vi "setup excel worksheet.vi"(0 "Current Sample Sheet":string="Sample 1", 1 "milliseconds to wait":u32=100, 3 "template file path":path=path "C:/Cascade/templates/Groundwater Profiling Log_empty_labview_template.xlsx", 4 "Excel report file path":path=path "C:/Cascade/Data/Excel Reports/Groundwater Profiling Log_ara1.xlsx", 5 "error in (no error)":errorcluster, 6 "Header path":path=path "C:/Cascade/templates/Fields for Excel sheets.xlsx", 7 "Open Excel Files":bool) -> (8 "subarray":string[][](array[string]), 10 "column max value":i32, 11 "row max value":i32, 12 "Column of Volume":i32, 13 "Worksheet Names":string[](array[string]), 14 "NI_report out":refnum<class "NI_report.lvclass">, 15 "Columns":i32[](array[numeric]), 16 "start of last occupied row":string, 17 "Number of Sample Sheets":i32, 18 "Select Worksheet Index":i32, 19 "error out":errorcluster)   [LabVIEW 2016]
uses:
  <vilib>/Utility/NIReport.llb/NI_report.lvclass
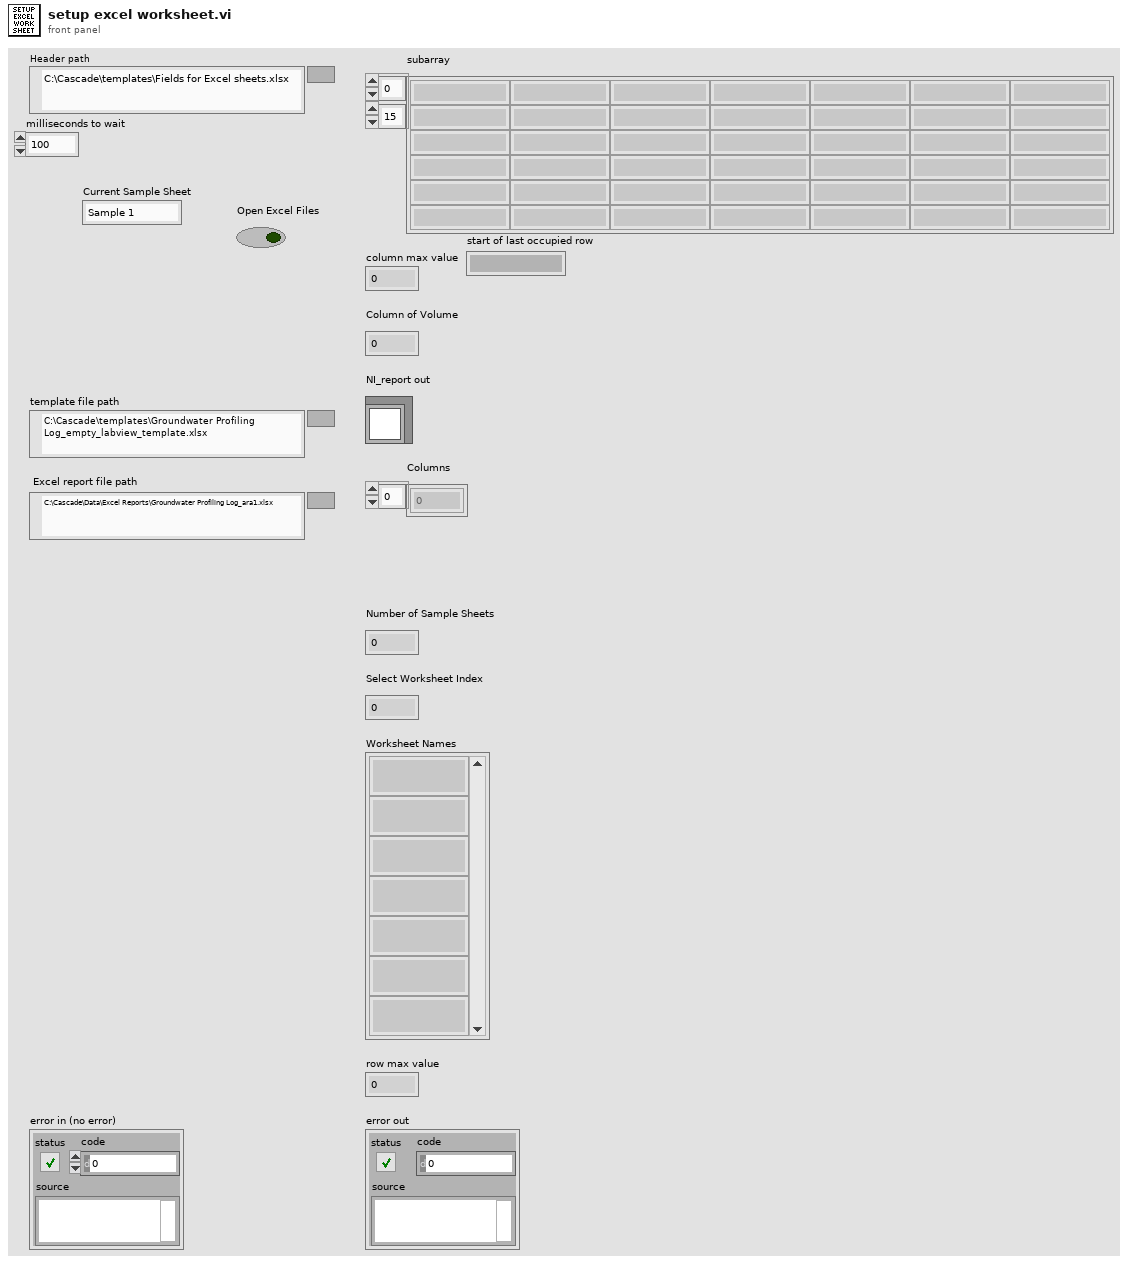
[diagram p1: front panel]
types:
  T1 = enum16{"maximized", "minimized", "normal", "no change"}
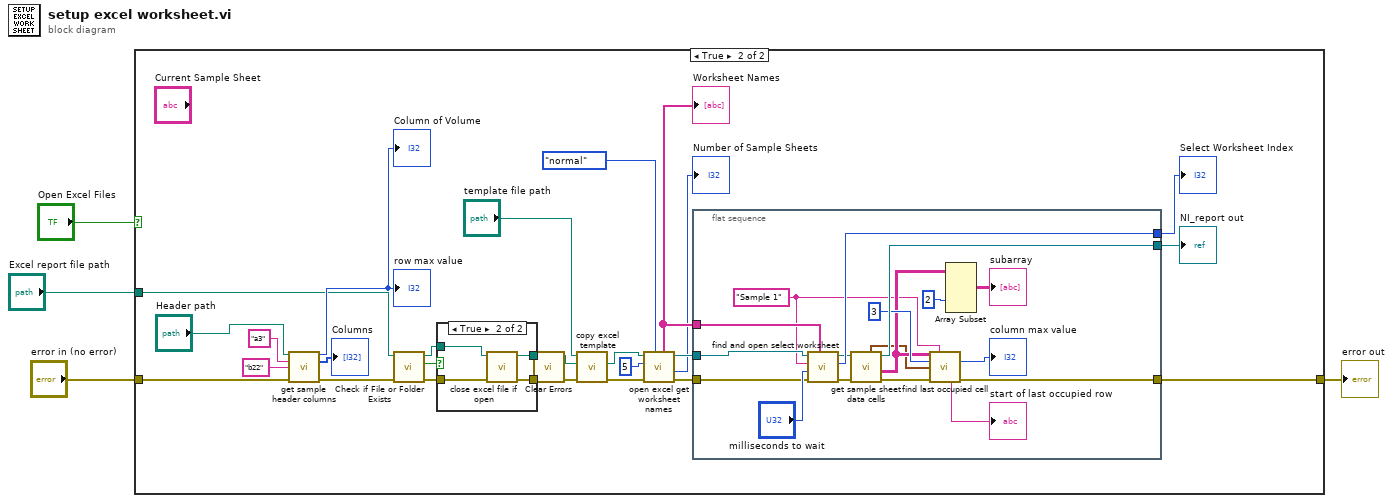
[diagram p0: block diagram]
diagram:
  n1 = case shown="True" "Open Excel Files" {
    tunnel: [_ w22] -> w4
    tunnel: "Excel report file path" -> [_ w9]
    tunnel: "error in (no error)" -> [_ w11]
    frame False {
    }
    frame True {
      n2 = call "get sample header columns.vi"("report file path"="Header path", "Start Cell Name"="a3", "Stop Cell name"="b22", "error in (no error)"=w11) -> ("Column of Volume"=→"row max value" →"Column of Volume":i32, "Columns"=→"Columns":i32[], "error out"=w10:errorcluster)  [unwired: 2 in, 7 out]
      n3 = call <vilib>:"Check if File or Folder Exists.vi"("error in (no error)"=w10, "path"=w9) -> ("error out"=w7:errorcluster, "file or folder exists?"=w6:bool, "dup path"=w8:path)  [unwired: 7 in]
      n4 = case shown="True" w6 {
        tunnel: [w31 w36] -> w23
        tunnel: [w32 w35] -> w16
        tunnel: w8 -> [w31 w34]
        tunnel: w7 -> [w32 w33]
        frame False {
        }
        frame True {
          n5 = call "close excel file if open.vi"("error in (no error)"=w33, "report file path in"=w34) -> ("error out"=w35:errorcluster, "report file path out"=w36:path)  [unwired: 8 in]
        }
      }
      n6 = call <vilib>:"Clear Errors.vi"("error in (no error)"=w16) -> ("error out"=w5:errorcluster)  [unwired: 5 in, 1 out]
      n7 = call "copy excel template.vi"("error in (no error)"=w5, "report file path in"=w23, "template file path in"="template file path") -> ("error out"=w15:errorcluster, "report file path out"=w13:path)  [unwired: 7 in]
      n8 = call "open excel get worksheet names.vi"("window state (normal)"=T1."normal", "error in (no error)"=w15, "milliseconds to wait"=u32 5, "report file path"=w13) -> ("error out"=w26:errorcluster, "Number of Sample Sheets"=→"Number of Sample Sheets":i32, "NI_report out"=w25:refnum<class "NI_report.lvclass">, "Worksheet Names"=w19:string[])  [unwired: 2 in, 2 out]
      "Worksheet Names" <- w19
      n9 = flat-sequence {
        tunnel: w19 -> [w53]
        tunnel: [w52] -> w20
        tunnel: [w50] -> w21
        tunnel: [w48] -> w22
        tunnel: w25 -> [w47]
        tunnel: w26 -> [w46]
        frame #0 {
          w37 = "Sample 1" ("Worksheet Name in")
          n10 = call "find and open select worksheet.vi"("Worksheet Names"=w53, "error in (no error)"=w46, "milliseconds to wait"="milliseconds to wait", "Worksheet Name in"=w37, "NI_report in"=w47) -> ("error out"=w49:errorcluster, "Select Worksheet Index"=w52:i32, "NI_report out"=w51:refnum<class "NI_report.lvclass">)  [unwired: 4 in]
          n11 = call "get sample sheet data cells.vi"("error in (no error)"=w49, "NI_report in"=w51) -> ("error out"=w42:errorcluster, "data"=w43:string[][], "NI_report out"=w50:refnum<class "NI_report.lvclass">, "left edge output cluster"=w41:cluster{"row":i32, "column":i32})  [unwired: 5 in, 1 out]
          n12 = call "find last occupied cell.vi"("data"=w43, "Active Sheet"=w37, "Header Rows to remove"=3, "sub array start"=w41, "error in (no error)"=w42) -> ("column max value"=→"column max value":i32, "start of last occupied row"=→"start of last occupied row":string, "error out"=w48:errorcluster)  [unwired: 4 in, 4 out]
          n13 = Array Subset(array=w43, index (col)=2 ("index")) -> (→"subarray":string[][])  [unwired: 3 in]
        }
      }
      "NI_report out" <- w21
      "Select Worksheet Index" <- w20
    }
  }
  "error out" <- w4
